vi "CTL_Spec LUTRev3.vi"(7 "Drain!Fill":bool, 8 "Level IN inches":dbl=5.0, 9 "Index":i32=3, 10 "ChA/!ChB":bool, 11 "Full Cfg":T3) -> (0 "Level Out":dbl, 1 "Set Point":dbl, 2 "Spec Range Out":T1, 3 "In Range?":bool=TRUE)   [LabVIEW 2024]
uses:
  Control Definitions/Def FullCfg.ctl
  Control Definitions/Def BenchCfg.ctl
  Control Definitions/Def PumpCtlRefs.ctl
  Control Definitions/Def_PumpSpeed.ctl
  Control Definitions/Def Bench Status.ctl
  Control Definitions/Def Spec RNG.ctl
  Control Definitions/Ded LUT_Status.ctl
panel:
  out "error out":errorcluster
  in  "error in (no error)":errorcluster
  # "In Range = TRUE when"
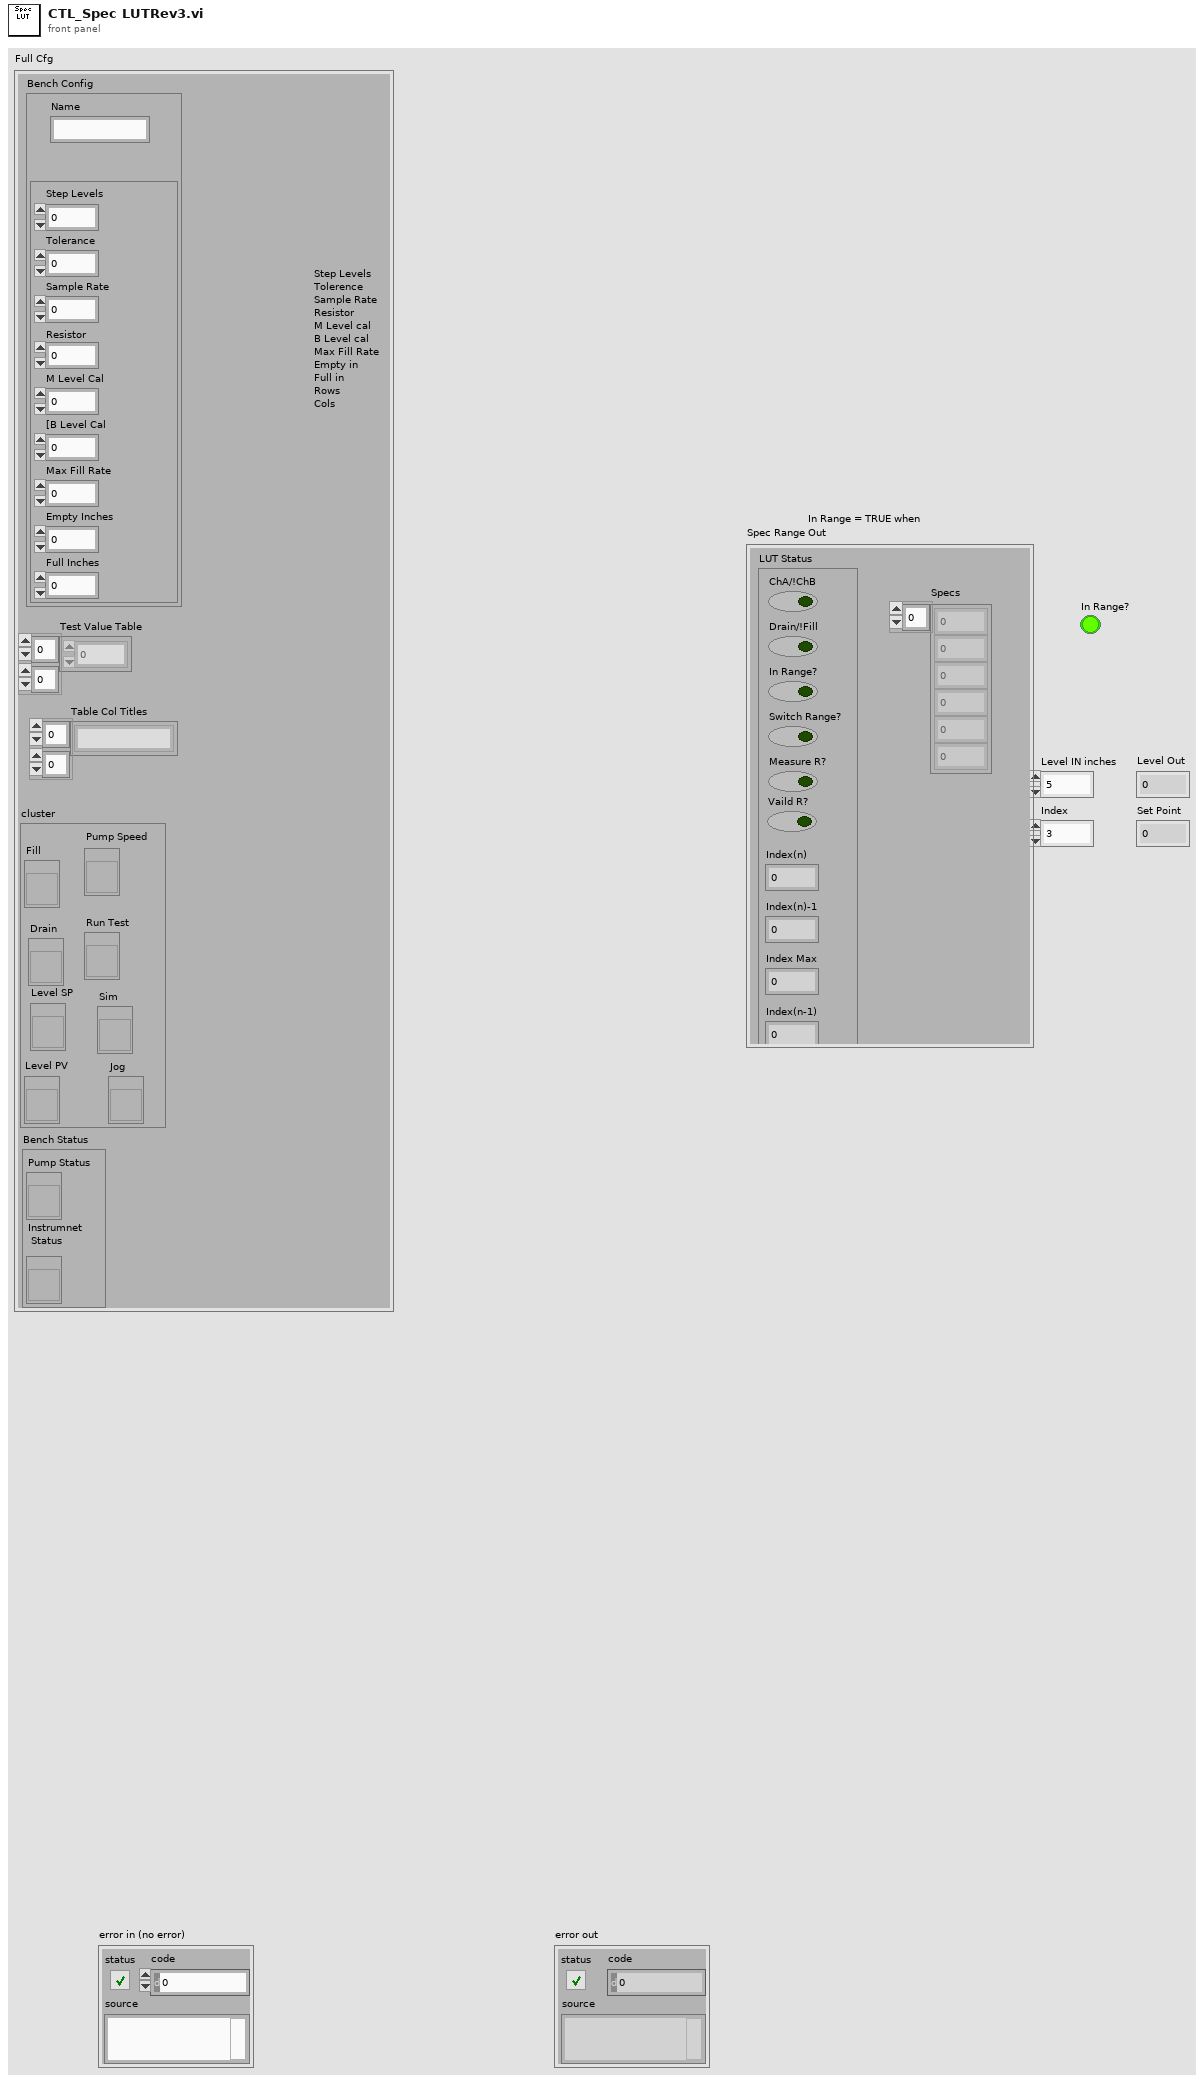
[diagram p1: front panel]
types:
  T1 = typedef "Def Spec RNG.ctl" = cluster{"Specs":dbl[], "LUT Status":T2}
  T2 = typedef "Ded LUT_Status.ctl" = cluster{"ChA/!ChB":bool, "Drain/!Fill":bool, "In Range?":bool, "Switch Range?":bool, "Measure R?":bool, "Vaild R?":bool, "Index(n)":i32, "Index(n)-1":i32, "Index Max":i32, "Index(n-1)":i32}
  T3 = typedef "Def FullCfg.ctl" = cluster{"Bench Config":T4, "Test Value Table ":dbl[][], "Table Col Titles":string[][], "cluster":T5, "Bench Status":T6}
  T4 = typedef "Def BenchCfg.ctl" = cluster{"Name":string, cluster{"Step Levels":dbl, "Tolerance":dbl, "Sample Rate":dbl, "Resistor":dbl, "M Level Cal":dbl, "[B Level Cal":dbl, "Max Fill Rate":dbl, "Empty Inches":dbl, "Full Inches":dbl}}
  T5 = typedef "Def PumpCtlRefs.ctl" = cluster{"Fill ":refnum<vi>, "Drain":refnum<vi>, "Level PV":refnum<vi>, "Pump Speed":refnum<vi>, "Run Test":refnum<vi>, "Sim":refnum<vi>, "Jog":refnum<vi>, "Level SP":refnum<vi>}
  T6 = typedef "Def Bench Status.ctl" = cluster{"Pump Status":refnum<vi>, "Instrumnet\n Status":refnum<vi>}
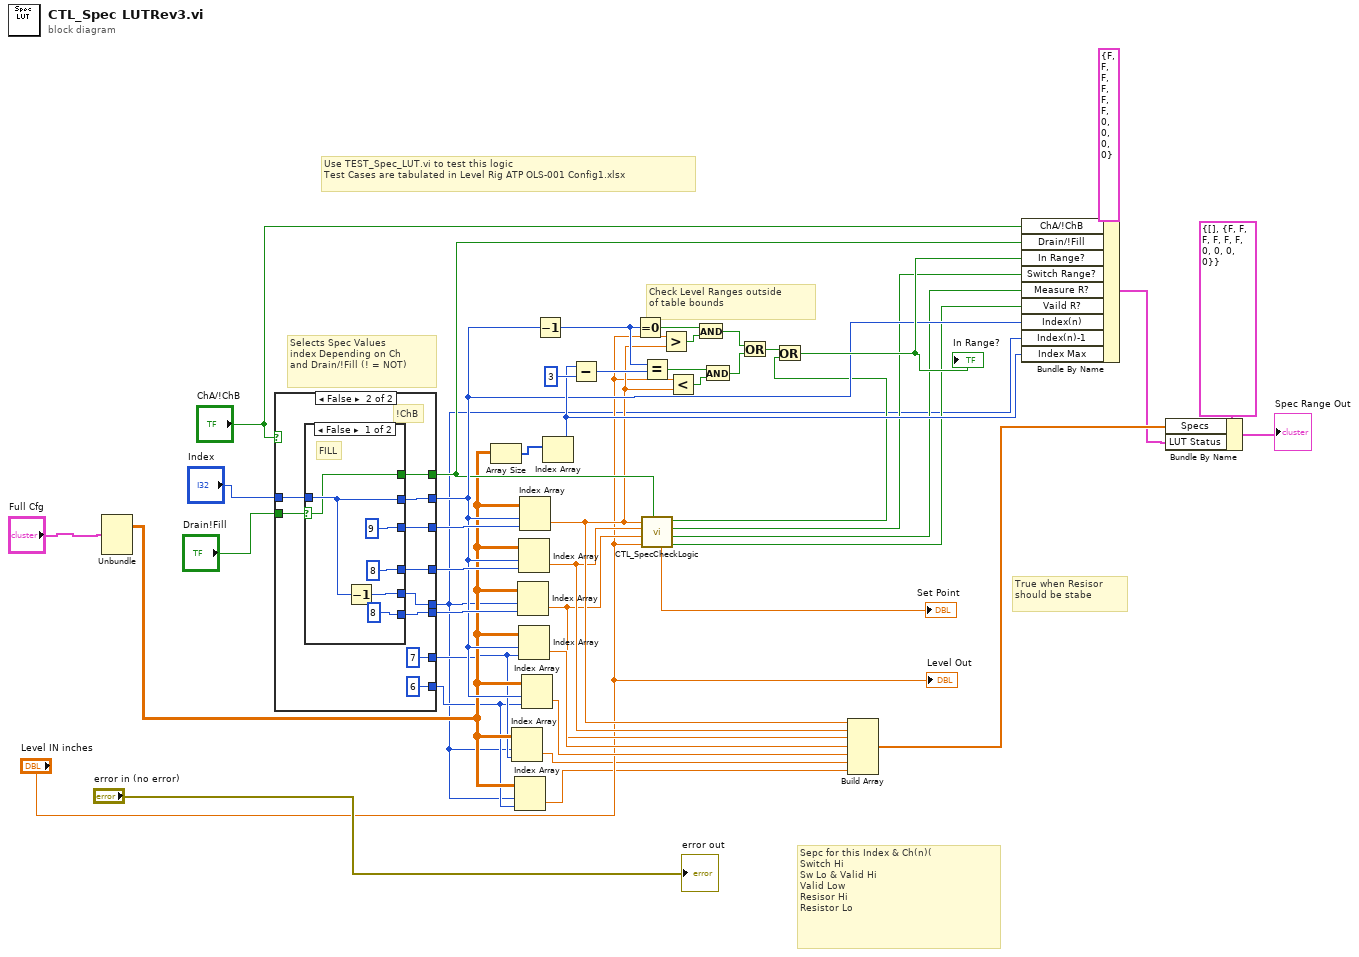
[diagram p0: block diagram]
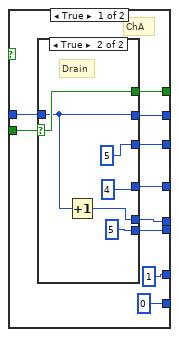
[diagram p2: hidden frame]
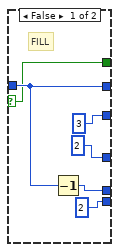
[diagram p3: hidden frame]
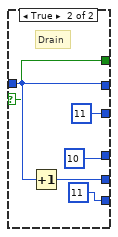
[diagram p4: hidden frame]
diagram:
  # "Use TEST_Spec_LUT.vi to test this logic\nTest Cases are tabulated in Level Rig ATP OLS-001 Config1.xlsx"
  # "Selects Spec Values\nindex Depending on Ch\nand Drain/!Fill (! = NOT)"
  # "True when Resisor \nshould be stabe"
  # "Sepc for this Index & Ch(n)(\nSwitch Hi\nSw Lo & Valid Hi  \nValid Low\nResisor Hi\nResistor Lo"
  # "Check Level Ranges outside \nof table bounds"
  n1 = Unbundle("Full Cfg") -> ("Test Value Table"=w6:dbl[][])  [unwired: 4 out]
  n2 = case shown="False" "ChA/!ChB" {
    tunnel: "Drain!Fill" -> [w55 w71]
    tunnel: "Index" -> [w54 w77]
    tunnel: [w53 w76] -> w17
    tunnel: [w52 w75] -> w3
    tunnel: [w51 w74] -> w44
    tunnel: [w50 w73] -> w43
    tunnel: [w49 w72] -> w30
    tunnel: [w48 w70] -> w16
    tunnel: [1 ("disabled index (col)") 7 ("disabled index (col)")] -> w5
    tunnel: [0 ("disabled index (col)") 6 ("disabled index (col)")] -> w4
    frame True {
      # "ChA"
      n3 = case shown="True" w55 {
        selector: w55 -> [w56 w64]
        tunnel: [2 ("disabled index (col)") 5 ("disabled index (col)")] -> w49
        tunnel: [3 ("disabled index (col)") 5 ("disabled index (col)")] -> w51
        tunnel: w54 -> [w57 w62]
        tunnel: [w57 w62] -> w53
        tunnel: [w59 w63] -> w52
        tunnel: [2 ("disabled index (col)") 4 ("disabled index (col)")] -> w50
        tunnel: [w56 w64] -> w48
        frame False {
          # "FILL"
          n4 = Decrement(x=w57) -> (x-1=w59:i32)
        }
        frame True {
          # "Drain"
          n5 = Increment(x=w62) -> (x+1=w63:i32)
        }
      }
    }
    frame False {
      # "!ChB"
      n6 = case shown="False" w71 {
        selector: w71 -> [w78 w84]
        tunnel: [8 ("disabled index (col)") 11 ("disabled index (col)")] -> w72
        tunnel: [9 ("disabled index (col)") 11 ("disabled index (col)")] -> w74
        tunnel: w77 -> [w79 w85]
        tunnel: [w79 w85] -> w76
        tunnel: [w81 w87] -> w75
        tunnel: [8 ("disabled index (col)") 10 ("disabled index (col)")] -> w73
        tunnel: [w78 w84] -> w70
        frame False {
          # "FILL"
          n7 = Decrement(x=w79) -> (x-1=w81:i32)
        }
        frame True {
          # "Drain"
          n8 = Increment(x=w85) -> (x+1=w87:i32)
        }
      }
    }
  }
  n9 = Array Size(array=w6) -> (size(s)=w28:i32[])
  n10 = Index Array(array=w6, index (row)=w3, index (col)=w5) -> (element=w2:dbl)
  n11 = Index Array(array=w6, index (row)=w3, index (col)=w4) -> (element=w1:dbl)
  n12 = Index Array(array=w6, index (row)=w3, index (col)=w30) -> (element=w13:dbl)
  n13 = Index Array(array=w6, index (row)=w17, index (col)=w43) -> (element=w14:dbl)
  n14 = Index Array(array=w6, index (row)=w17, index (col)=w5) -> (element=w42:dbl)
  n15 = Index Array(array=w6, index (row)=w17, index (col)=w44) -> (element=w15:dbl)
  n16 = Index Array(array=w6, index (row)=w17, index (col)=w4) -> (element=w41:dbl)
  n17 = Decrement(x=w17) -> (x-1=w21:i32)
  n18 = Index Array(array=w28) -> (element=w18:i32)  [unwired: 1 in]
  n19 = Subtract(x=w18, y=3) -> (x-y=w26:i32)
  n20 = Equal To 0?(x=w21) -> (x = 0?=w37:bool)
  n21 = Equal?(x=w21, y=w26) -> (x = y?=w39:bool)
  n22 = call "CTL_SpecCheckLogic.vi"("Drain!Fill In"=w16, "Level in"="Level IN inches", "Spec Hi(n+1)"=w13, "Spec Lo (n)"=w14, "Spec Hi (n)"=w15) -> ("Vaild R?"=w8:bool, "Measure R?"=w7:bool, "Switch Range?"=w10:bool, "In Range?"=w11:bool, "Set Point"=→"Set Point":dbl)  [unwired: 2 in]
  n23 = Greater?(x="Level IN inches", y=w15) -> (0:w38:bool)
  n24 = Less?(x="Level IN inches", y=w15) -> (x < y?=w40:bool)
  n25 = And(x=w37, y=w38) -> (x .and. y?=w35:bool)
  n26 = And(x=w39, y=w40) -> (x .and. y?=w36:bool)
  n27 = Or(x=w35, y=w36) -> (x .or. y?=w34:bool)
  n28 = Or(x=w34, y=w11) -> (x .or. y?=w25:bool)
  "In Range?" <- w25
  n29 = Build Array(w15, w14, w13, w42, w41, w2, w1) -> (w24:dbl[])
  n30 = Bundle By Name(cluster=T2 {"ChA/!ChB"=FALSE, "Drain/!Fill"=FALSE, "In Range?"=FALSE, "Switch Range?"=FALSE, "Measure R?"=FALSE, "Vaild R?"=FALSE, "Index(n)"=0, "Index(n)-1"=0, "Index Max"=0, "Index(n-1)"=0} ("LUT Status Def"), "ChA/!ChB"="ChA/!ChB", "Drain/!Fill"=w16, "In Range?"=w25, "Switch Range?"=w10, "Measure R?"=w7, "Vaild R?"=w8, "Index(n)"=w17, "Index(n)-1"=w3, "Index Max"=w18) -> (w20:T2)
  n31 = Bundle By Name(cluster=T1 {"Specs"=[], "LUT Status"={"ChA/!ChB"=FALSE, "Drain/!Fill"=FALSE, "In Range?"=FALSE, "Switch Range?"=FALSE, "Measure R?"=FALSE, "Vaild R?"=FALSE, "Index(n)"=0, "Index(n)-1"=0, "Index Max"=0, "Index(n-1)"=0}} ("Spec Raange Def"), "Specs"=w24, "LUT Status"=w20) -> (→"Spec Range Out":T1)
  "error out" <- "error in (no error)"
  "Level Out" <- "Level IN inches"
